vi "Close_all_queues.vi"(11 "Process queues":refnum<queue>[](array[refnum])) -> ()   [LabVIEW 2017, in "labview-standard-library.lvlib" / "automode-scripting.lvlib"]
uses:
  automode-scripting.lvlib
  type-defs/command_line_info.ctl
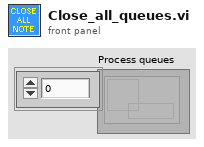
[diagram p1: front panel]
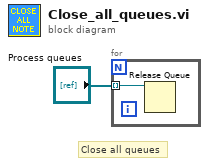
[diagram p0: block diagram]
diagram:
  # "Close all queues"
  n1 = for {
    tunnel: "Process queues" -> [w2] mode=indexing
    n2 = Release Queue(queue=w2) -> ()  [unwired: 2 in, 3 out]
  }
